vi "gratings_and_lenses_with_feedback.vi"(2 "Resolution":i32, 3 "Spots 2":T1[](array[typedef]) {"Amplitude Correction" step=0.1; "Line Trapping"."Phase Gradient" step=0.05; "Line Trapping"."Vector"."x" step=1e-06 format="%#_6p"; "Line Trapping"."Vector"."y" step=1e-06 format="%#_6p"; "Line Trapping"."Vector"."z" step=1e-06 format="%#_6p"; "NA Position"."r" step=1e-06; "NA Position"."y" step=1e-06; "NA Position"."x" step=1e-06; "Position"."z" step=1e-06; "Position"."y" step=1e-06; "Position"."x" step=1e-06; "Phase" step=0.7753; "Intensity" step=0.1}) -> (0 "Spot Amplitudes":cdb[](array[numeric]), 1 "Complex Hologram":cdb[][](array[numeric]))   [LabVIEW 2019]
uses:
  spot.ctl
  line_trapping.ctl
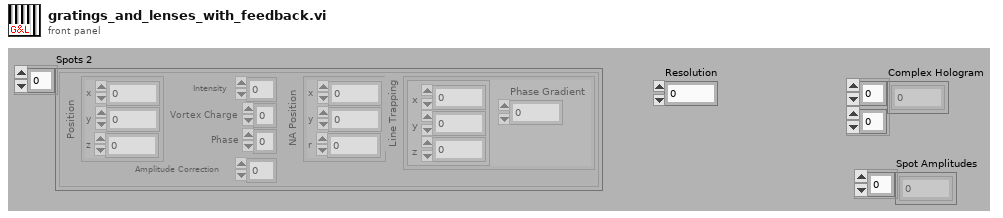
[diagram p1: front panel]
types:
  T1 = typedef "spot.ctl" = cluster{"Position":cluster{"x":dbl, "y":dbl, "z":dbl}, "Intensity":dbl, "Vortex Charge":i8, "Phase":dbl, "NA Position":cluster{"x":dbl, "y":dbl, "r":dbl}, "Line Trapping":T2, "Amplitude Correction":dbl}
  T2 = typedef "line_trapping.ctl" = cluster{"Vector":cluster{"x":dbl, "y":dbl, "z":dbl}, "Phase Gradient":dbl}
  T3 = cluster{"X tilt":dbl, "Y tilt":dbl, "Z shift":dbl, "L (vortex)":dbl, "Phase":dbl, "Amplitude":dbl, "Corrector":dbl}
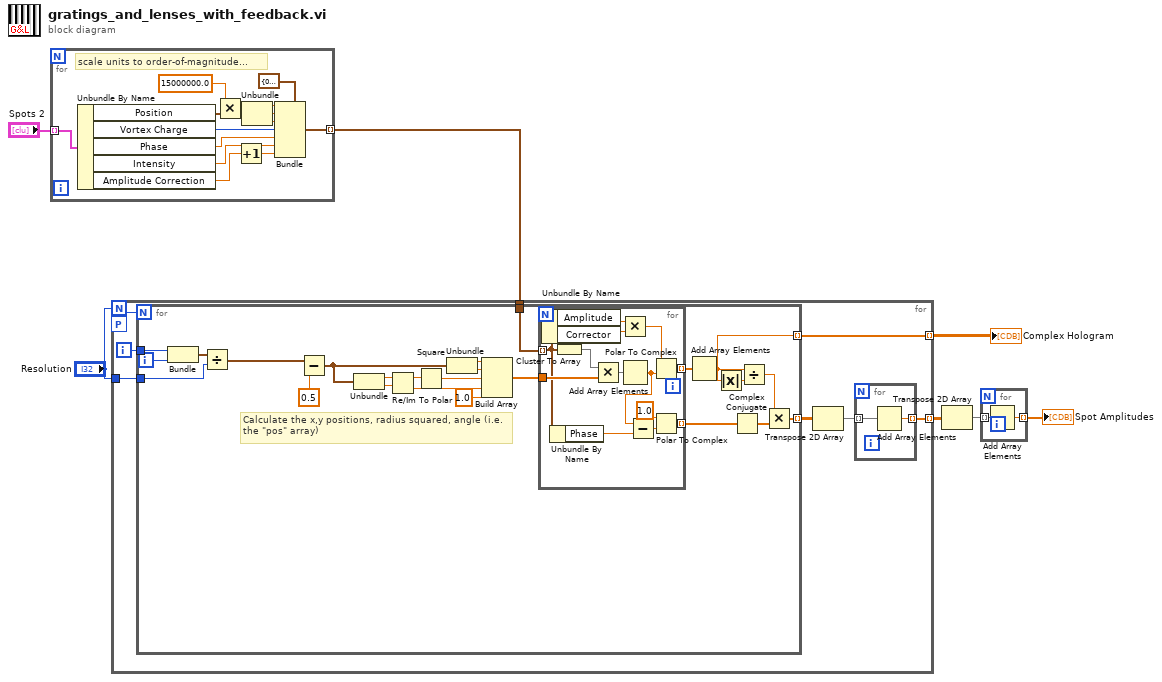
[diagram p0: block diagram]
diagram:
  n1 = for {
    tunnel: "Spots 2" -> [w21] mode=indexing
    tunnel: [w17] -> w1 mode=indexing
    # "scale units to order-of-magnitude..."
    n2 = Unbundle By Name(w21) -> ("Position"=w16:cluster{"x":dbl, "y":dbl, "z":dbl}, "Vortex Charge"=w20:i8, "Phase"=w19:dbl, "Intensity"=w18:dbl, "Amplitude Correction"=w9:dbl)
    n3 = Multiply(x=15000000.0 ("Phase"), y=w16) -> (x*y=w14:cluster{"x":dbl, "y":dbl, "z":dbl})
    n4 = Increment(x=w9) -> (x+1=w8:dbl)
    n5 = Unbundle(w14) -> ("x"=w13:dbl, "y"=w12:dbl, "z"=w11:dbl)
    n6 = Bundle(cluster=T3 {"X tilt"=0.0, "Y tilt"=0.0, "Z shift"=0.0, "L (vortex)"=0.0, "Phase"=0.0, "Amplitude"=0.0, "Corrector"=0.0} ("Spot"), "X tilt"=w13, "Y tilt"=w12, "Z shift"=w11, "L (vortex)"=w20, "Phase"=w19, "Amplitude"=w18, "Corrector"=w8) -> (w17:T3)
  }
  n7 = for {
    N: "Resolution" -> [w29]
    tunnel: "Resolution" -> [w27]
    tunnel: w1 -> [w26]
    workers-P: _ -> [_]
    tunnel: [w23] -> w3 mode=indexing
    tunnel: [w22] -> w6 mode=indexing
    i -> [w28]
    n8 = for {
      N: w29 -> [_]
      tunnel: w28 -> [w54]
      tunnel: w27 -> [w53]
      tunnel: w26 -> [w50]
      tunnel: [w39] -> w25 mode=indexing
      tunnel: [w33] -> w22 mode=indexing
      i -> [w55]
      # "Calculate the x,y positions, radius squared, angle (i.e. the \"pos\" array)"
      n9 = Bundle(w54, w55) -> (w32:cluster{i32, i32})  [unwired: 1 in]
      n10 = Divide(x=w32, y=w53) -> (x/y=w49:cluster{dbl, dbl})
      n11 = Subtract(x=w49, y=0.5) -> (x-y=w41:cluster{dbl, dbl})
      n12 = Unbundle(w41) -> (w47:dbl, w46:dbl)
      n13 = Re/Im To Polar(2:w46, 3:w47) -> (0:w43:dbl, 1:w44:dbl)
      n14 = Square(x=w44) -> (x^2=w45:dbl)
      n15 = Unbundle(w41) -> (w52:dbl, w51:dbl)
      n16 = Build Array(w52, w51, w45, w43, sgl 1.0 ("element")) -> (w38:dbl[])
      n17 = for {
        tunnel: w38 -> [w68]
        tunnel: w50 -> [w59] mode=indexing
        tunnel: [w66] -> w40 mode=indexing
        tunnel: [w60] -> w36 mode=indexing
        n18 = Unbundle By Name(w59) -> ("Amplitude"=w64:dbl, "Corrector"=w62:dbl)
        n19 = Unbundle By Name(w59) -> ("Phase"=w57:dbl)
        n20 = Cluster To Array(cluster=w59) -> (array=w65:dbl[])
        n21 = Multiply(x=w65, y=w68) -> (x*y=w67:dbl[])
        n22 = Multiply(x=w64, y=w62) -> (x*y=w63:dbl)
        n23 = Add Array Elements(numeric array=w67) -> (sum=w56:dbl)
        n24 = Subtract(x=w56, y=w57) -> (x-y=w58:dbl)
        n25 = Polar To Complex(1:w56, 2:w63) -> (0:w66:cdb)
        n26 = Polar To Complex(1:w58, 2:1.0 ("r")) -> (0:w60:cdb)
      }
      n27 = Add Array Elements(numeric array=w40) -> (sum=w33:cdb)
      n28 = Absolute Value(x=w33) -> (abs(x)=w34:dbl)
      n29 = Complex Conjugate(1:w36) -> (0:w37:cdb[])
      n30 = Divide(x=w33, y=w34) -> (x/y=w35:cdb)
      n31 = Multiply(x=w35, y=w37) -> (x*y=w39:cdb[])
    }
    n32 = Transpose 2D Array(2D array=w25) -> (transposed array=w24:cdb[][])
    n33 = for {
      tunnel: w24 -> [w31] mode=indexing
      tunnel: [w30] -> w23 mode=indexing
      n34 = Add Array Elements(numeric array=w31) -> (sum=w30:cdb)
    }
  }
  "Complex Hologram" <- w6
  n35 = Transpose 2D Array(2D array=w3) -> (transposed array=w4:cdb[][])
  n36 = for {
    tunnel: w4 -> [w70] mode=indexing
    tunnel: [w69] -> w5 mode=indexing
    n37 = Add Array Elements(numeric array=w70) -> (sum=w69:cdb)
  }
  "Spot Amplitudes" <- w5
